vi "epx_Update Vector Size.vi"(7 "Container State":T1, 8 "error in (no error)":errorcluster, 9 "Background Decoratin":refnum<vi>, 10 "Display State In":T2={"BGColor"=0, "FGColor"=0, "GridColor"=9868950, "Number of Polar Grids"=12, "Number of Circle Grids"=4, "Vector.Active"=0, "Vectors.Properties"=[], "Height"=0, "Width"=0} {"Number of Circle Grids" min=1 max=100 step=1; "Number of Polar Grids" min=1 max=100 step=1}, 11 "Vector Diagram":refnum<vi>) -> (0 "error out":errorcluster, 1 "Background Decoratin out":refnum<vi>, 3 "Vector Diagram out":refnum<vi>)   [LabVIEW 2011, in "NI_EP_Basic.lvlib" / "EPX Vector Diagram.xctl"]
uses:
  <vilib>/addons/Electrical Power/Basic/Controls/Vector Diagram/Abilities/epx_Vector Diagram State.ctl
  <vilib>/addons/Electrical Power/Basic/Controls/Vector Diagram/SubVIs/epx_Vector Type.ctl
  <vilib>/_xctls/Container State.ctl
  <vilib>/Utility/miscctls.llb/LVPositionTypeDef.ctl
  <vilib>/Utility/miscctls.llb/LVBoundsTypeDef.ctl
  <vilib>/addons/Electrical Power/Basic/Controls/Vector Diagram/EPX Vector Diagram.xctl
  <vilib>/addons/Electrical Power/Basic/NI_EP_Basic.lvlib
  <vilib>/_xctls/XControlSupport.lvlib
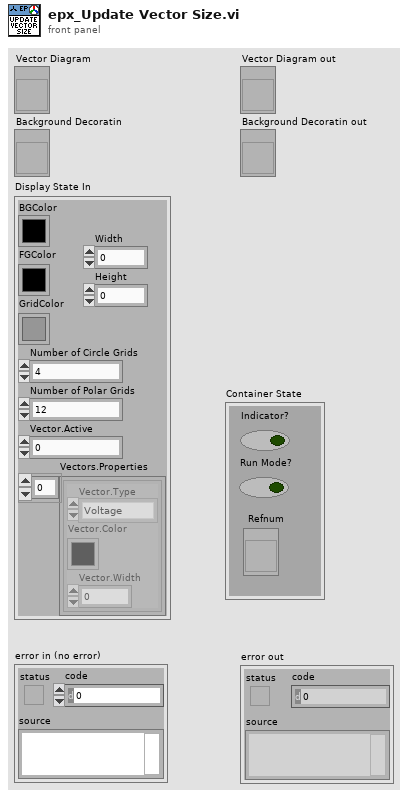
[diagram p1: front panel]
types:
  T1 = typedef "XControlSupport.lvlib/Container State.ctl" = cluster{"Indicator?":bool, "Run Mode?":bool, " Refnum":refnum<vi>}
  T2 = typedef "NI_EP_Basic.lvlib/EPX Vector Diagram.xctl/epx_Vector Diagram State.ctl" = cluster{"BGColor":u32, "FGColor":u32, "GridColor":u32, "Number of Polar Grids":i32, "Number of Circle Grids":i32, "Vector.Active":i32, "Vectors.Properties":cluster{"Vector.Type":T3, "Vector.Color":u32, "Vector.Width":u8}[], "Height":u32, "Width":u32}
  T3 = typedef "NI_EP_Basic.lvlib/epx_Vector Type.ctl" = enum16{"Voltage", "Current"}
  T4 = cluster{"BGColor":bool, "FGColor":bool, "GridColor":bool, "Number of Polar Grids":bool, "Number of Circle Grids":bool, "Vector.Active":bool, "Vectors.Properties":cluster{"Vector.Type":bool, "Vector.Color":bool, "Vector.Width":bool}[], "Height":bool, "Width":bool}
  T5 = typedef "LVPositionTypeDef.ctl" = cluster{"Left":i32, "Top":i32}
  T6 = typedef "LVBoundsTypeDef.ctl" = cluster{"Width":u32, "Height":u32}
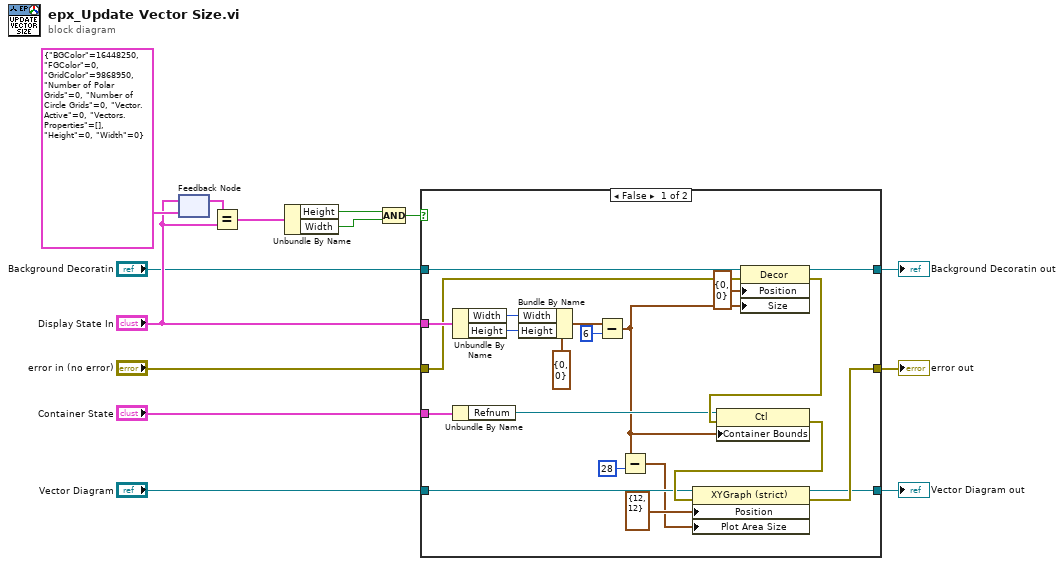
[diagram p0: block diagram]
diagram:
  n1 = feedback-in #1("Display State In") -> ()
  n2 = feedback #1(T2 {"BGColor"=16448250, "FGColor"=0, "GridColor"=9868950, "Number of Polar Grids"=0, "Number of Circle Grids"=0, "Vector.Active"=0, "Vectors.Properties"=[], "Height"=0, "Width"=0} ("Display State In")) -> (w10:T2)
  n3 = Equal?(x=w10, y="Display State In") -> (x = y?=w9:T4)
  n4 = Unbundle By Name(w9) -> ("Height"=w5:bool, "Width"=w4:bool)
  n5 = Compound Arithmetic op=AND(w5, w4) -> (w8:bool)
  n6 = case shown="False" w8 {
    tunnel: [w27 w37] -> w14
    tunnel: [w26 w38] -> w13
    tunnel: "Vector Diagram" -> [w28 w38]
    tunnel: "error in (no error)" -> [w31 w37]
    tunnel: "Display State In" -> [w32 _]
    tunnel: "Background Decoratin" -> [w30 w36]
    tunnel: "Container State" -> [w29 _]
    tunnel: [w25 w36] -> w1
    frame False {
      n7 = Unbundle By Name(w32) -> ("Width"=w20:u32, "Height"=w19:u32)
      n8 = Unbundle By Name(w29) -> ("Refnum"=w33:refnum<vi>)
      n9 = Bundle By Name(cluster=T6 {"Width"=0, "Height"=0} ("XControl:Container Bounds"), "Width"=w20, "Height"=w19) -> (w17:T6)
      n10 = Subtract(x=w17, y=u32 6) -> (x-y=w16:T6)
      n11 = Subtract(x=w16, y=u32 28) -> (x-y=w15:T6)
      n12 = property class="Decor"(reference=w30, error in=w31, "Position"=T5 {"Left"=0, "Top"=0}, "Size"=w16) -> (reference out=w25:refnum<vi>, error out=w34:errorcluster)
      n13 = property class="Ctl"(reference=w33, error in=w34, "Container Bounds"=w16) -> (error out=w35:errorcluster)  [unwired: 1 out]
      n14 = property on="Property Node" class="XYGraph (strict)"(reference=w28, error in=w35, "Position"=T5 {"Left"=12, "Top"=12}, "Plot Area Size"=w15) -> (reference out=w26:refnum<vi>, error out=w27:errorcluster)
    }
    frame True {
    }
  }
  "error out" <- w14
  "Vector Diagram out" <- w13
  "Background Decoratin out" <- w1
